vi "RT Analysis Workspace.vi"() -> ()   [LabVIEW 2023]
doc: "This example demonstrates the use of the Real-Time Analysis Utilities VIs to reduce jitter in Mathematics and Signal Processing VIs running on RT targets. The VI also compares the execution time of analysis VIs when used with the Real-Time Analysis Utilities VIs to the execution time of analysis VIs when used without the Real-Time Analysis Utilities VIs. This example is intended for use with the ETS real-time operating system."
uses:
  <vilib>/Platform/TimedLoop/XDataNode/timing_clust.ctl
  <vilib>/Platform/TimedLoop/XDataNode/nitl_modes.ctl
  <vilib>/Platform/TimedLoop/XDataNode/wakeup.ctl
  <vilib>/Platform/TimedLoop/XDataNode/XDataNode.xnode
  <vilib>/Analysis/NI_AALPro.lvlib
  <vilib>/Platform/TimedLoop/XDataNode/XDNodeRunTimeDep.lvlib
panel:
  in  "Stop":bool
  out "Mean Time (Normal Execution)":dbl
  out "Max Jitter (Normal Execution)":dbl
  out "Max Jitter (Analysis Workspace)":dbl
  out "Mean Time (Analysis Workspace)":dbl
  in  "Warmup Iterations":i32=10
  in  "Iterations":i32=1000
  out "Execution Time (us)":u32[][](graph)
  # "Overview: This example demonstrates the use of the Real-Time Analysis Workspace VIs to reduce jitter in Mathematics and Signal Processing VIs running on LabVIEW Real-Time targets.\nRequirements: LabVIEW Full Development System, LabVIEW Real-Time Module\nInstructions:\n1. Select the number of iterations to run and the number of warmup iterations to exclude from the benchmark.\n2. Run the VI.\n3. Compare the execution times of the analysis VIs running with the Real-Time Analysis Workspace VIs versus normal execution. View the block diagram to see how you can use the Real-Time Analysis Workspace VIs to reduce the effects of jitter."
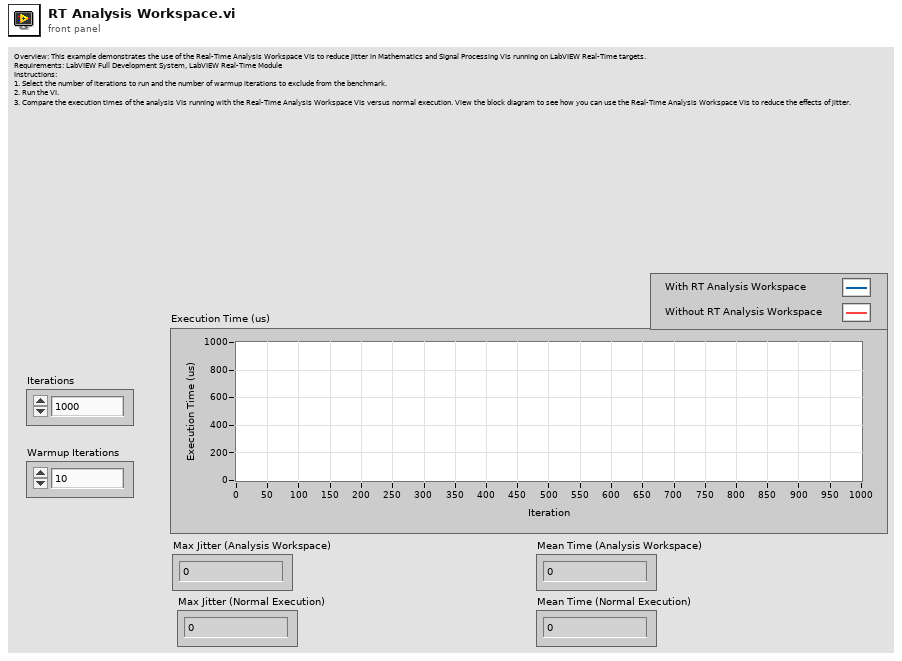
[diagram p1: front panel]
types:
  T1 = typedef "XDNodeRunTimeDep.lvlib/timing_clust.ctl" = cluster{"Expected End [f-1]":u64, "Actual End [f-1]":u64, "Finished Late? [f-1]":bool, "Expected End [i-1]":u64, "Actual End [i-1]":u64, "Finished Late? [i-1]":bool, "Expected Start [i]":u64, "Actual Start [i]":u64, "Expected Start [f]":u64, "Actual Start [f]":u64, "Source Name":string, "Structure Name":string, "Period":i64, "Deadline":i64, "Offset":i64, "Start":i64, "Priority":i32, "Timeout":i32, "Mode":T2, "Wakeup Reason":T3, "Error":errorcluster, "Source Type":string, "Secondary Source Type":string, "Global End Time":u64, "Global Start Time":u64, "Frame Duration":u64, "Iteration Duration":u64, "Assigned CPU":i32, "I/O Scan Engine Mode":u32}
  T2 = typedef "XDNodeRunTimeDep.lvlib/nitl_modes.ctl" = enum32{"No Change", "Process missed periods, maintain original phase", "Discard missed periods, maintain original phase", "Process missed periods, ignore original phase", "Discard missed periods, ignore original phase"}
  T3 = typedef "XDNodeRunTimeDep.lvlib/wakeup.ctl" = enum32{"Normal", "Aborted", "Asynchronous wakeup", "Timing source error", "Timed loop error", "Timeout"}
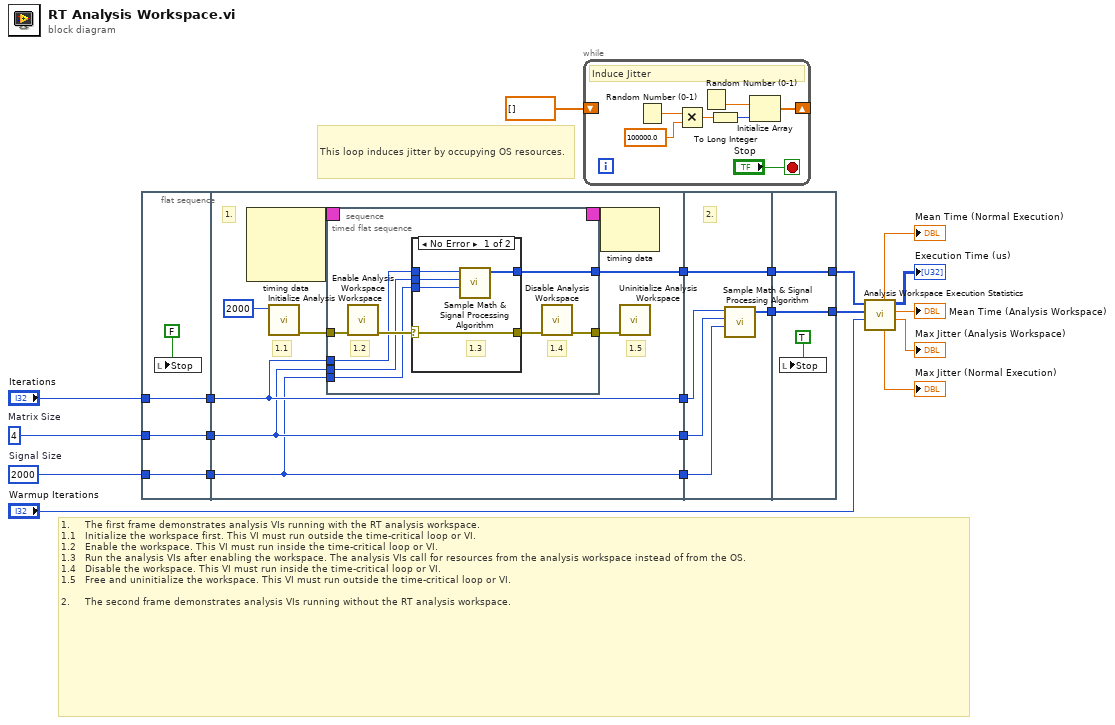
[diagram p0: block diagram]
diagram:
  w2 = 2000  # Signal Size
  w5 = 4  # Matrix Size
  # "1.     The first frame demonstrates analysis VIs running with the RT analysis workspace.\n1.1   Initialize the workspace first. This VI must run outside the time-critical loop or VI.\n1.2   Enable the workspace. This VI must run inside the time-critical loop or VI.\n1.3   Run the analysis VIs after enabling the workspace. The analysis VIs call for resources from the analysis workspace instead of from the OS.\n1.4   Disable the workspace. This VI must run inside the time-critical loop or VI.\n1.5   Free and uninitialize the workspace. This VI must run outside the time-critical loop or VI.\n\n2.     The second frame demonstrates analysis VIs running without the RT analysis workspace."
  # "This loop induces jitter by occupying OS resources."
  n1 = flat-sequence {
    tunnel: [w24] -> w9
    tunnel: "Iterations" -> [w24]
    tunnel: [w23] -> w6
    tunnel: w5 -> [w23]
    tunnel: [w22] -> w3
    tunnel: w2 -> [w22]
    tunnel: [w29] -> w15
    tunnel: w9 -> [w28]
    tunnel: [w28] -> w7
    tunnel: w6 -> [w27]
    tunnel: [w27] -> w4
    tunnel: w3 -> [w26]
    tunnel: [w26] -> w1
    tunnel: w15 -> [w63]
    tunnel: [w63] -> w13
    tunnel: [w62] -> w12
    tunnel: w7 -> [w61]
    tunnel: w4 -> [w60]
    tunnel: w1 -> [w59]
    tunnel: [w65] -> w14
    tunnel: [w66] -> w20
    tunnel: w13 -> [w66]
    tunnel: w12 -> [w65]
    frame #0 {
      n2 = local write "Stop"(FALSE) -> ()
    }
    frame #1 {
      # "1.5"
      # "1.1"
      # "1."
      n3 = node-c288() -> (w34:T1)  [unwired: 3 in]
      n4 = call <vilib>:"Initialize Analysis Workspace.vi"("reserved memory size (KB)"=u32 2000) -> ("error out"=w32:errorcluster)  [unwired: 10 in]
      n5 = timed-sequence {
        timing: w34 -> [_]
        timing-out: [_] -> w33
        tunnel: w32 -> [w40]
        tunnel: [w39] -> w31
        tunnel: [w38] -> w29
        tunnel: w28 -> [w37]
        tunnel: w27 -> [w36]
        tunnel: w26 -> [w35]
        n6 = timed-flat-sequence {
          tunnel: w40 -> [w48]
          tunnel: [w46] -> w38
          tunnel: [w47] -> w39
          tunnel: w37 -> [w43]
          tunnel: w36 -> [w42]
          tunnel: w35 -> [w41]
          # "1.4"
          # "1.2"
          n7 = call <vilib>:"Enable Analysis Workspace.vi"("error in (no error)"=w48) -> ("error out"=w45:errorcluster)  [unwired: 10 in]
          n8 = case shown="No Error" w45 {
            selector: w45 -> [w53 w54]
            tunnel: [w52 _] -> w46
            tunnel: [w53 w54] -> w44
            tunnel: w43 -> [w51 _]
            tunnel: w42 -> [w50 _]
            tunnel: w41 -> [w49 _]
            frame No Error {
              # "1.3"
              n9 = call "Sample Math & Signal Processing Algorithm.vi"("signal size"=w49, "matrix size"=w50, "iteration"=w51) -> ("Time Per Iteration"=w52:u32[])  [unwired: 7 in, 1 out]
            }
            frame Error {
            }
          }
          n10 = call <vilib>:"Disable Analysis Workspace.vi"("error in (no error)"=w44) -> ("error out"=w47:errorcluster)  [unwired: 10 in]
        }
      }
      n11 = node-c288(w33) -> ()  [unwired: 1 out]
      n12 = call <vilib>:"Uninitialize Analysis Workspace.vi"("error in (no error)"=w31) -> ()  [unwired: 10 in, 1 out]
    }
    frame #2 {
      # "2."
      n13 = call "Sample Math & Signal Processing Algorithm.vi"("signal size"=w59, "matrix size"=w60, "iteration"=w61) -> ("Time Per Iteration"=w62:u32[])  [unwired: 7 in, 1 out]
    }
    frame #3 {
      n14 = local write "Stop"(TRUE) -> ()
    }
  }
  n15 = while {
    shift-right: [w73] -> _
    shift-left: dbl[] [] -> [_]
    stop <- "Stop" stop-if-true
    # "Induce Jitter"
    n16 = Random Number (0-1)() -> (number: 0 to 1=w71:dbl)
    n17 = Multiply(x=w71, y=100000.0) -> (x*y=w69:dbl)
    n18 = Random Number (0-1)() -> (number: 0 to 1=w72:dbl)
    n19 = To Long Integer(number=w69) -> (32bit integer=w68:i32)
    n20 = Initialize Array(w72, w68) -> (w73:dbl[])
  }
  n21 = call "Analysis Workspace Execution Statistics.vi"("Warmup Iterations"="Warmup Iterations", "Time Per Iteration 2"=w14, "Time Per Iteration"=w20) -> ("Max Jitter"=→"Max Jitter (Analysis Workspace)":dbl, "Mean Time"=→"Mean Time (Analysis Workspace)":dbl, "Execution Time"=→"Execution Time (us)":u32[][], "Max Jitter 2"=→"Max Jitter (Normal Execution)":dbl, "Mean Time 2"=→"Mean Time (Normal Execution)":dbl)  [unwired: 4 in]
